vi "VI-Create XControl Dialog.vi"() -> ()   [LabVIEW 2015]
panel:
  out "exit":bool
  in  "XControl":cluster{"Folder":path, "Name":string}={"Folder"=path "D:/Experiment VIs", "Name"="New XControl"}
  in  "Create XControl":bool
  # "XControl"
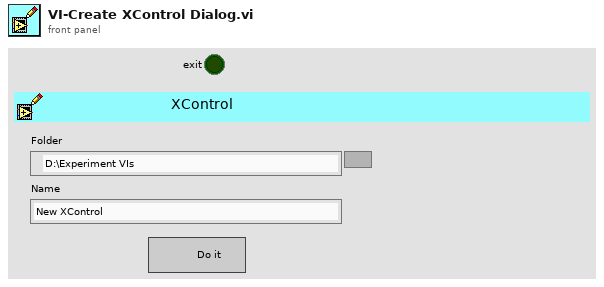
[diagram p1: front panel]
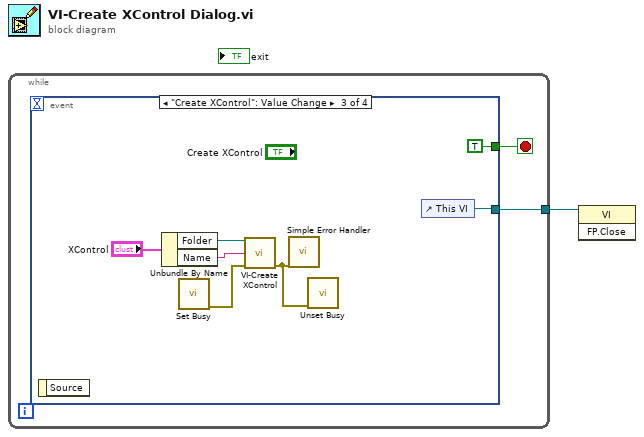
[diagram p0: block diagram]
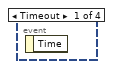
[diagram p2: hidden frame]
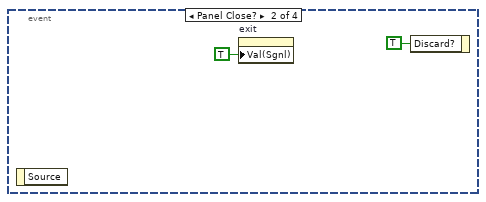
[diagram p3: hidden frame]
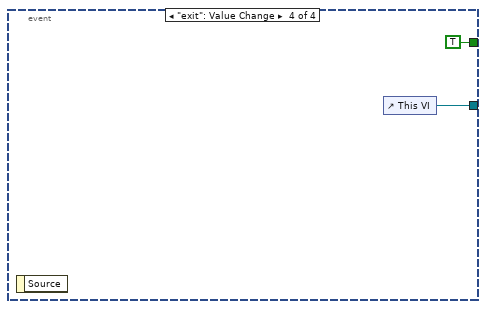
[diagram p4: hidden frame]
diagram:
  n1 = while {
    tunnel: [w3] -> w1
    stop <- w2 stop-if-true
    n2 = event shown="[2] \"Create XControl\": Value Change" {
      selector: _ -> [_ _ _ _]
      dyn-events: _ -> [_ _ _ _]
      timeout: _ -> [_ _ _ _]
      tunnel: [_ _ w8 w14] -> w3
      tunnel: [_ _ TRUE TRUE] -> w2
      event Timeout {
        n3 = event-data() -> ()  [unwired: 1 in, 1 out]
      }
      event Panel Close? {
        n4 = event-data() -> ()  [unwired: 1 in, 1 out]
        n5 = property on="exit" class="Bool (strict)"("Val(Sgnl)"=TRUE ("Value (Signaling)")) -> ()  [unwired: 2 in, 2 out]
        n6 = event-data("Discard?"=TRUE) -> ()  [unwired: 1 in, 1 out]
      }
      event "Create XControl": Value Change {
        n7 = event-data() -> ()  [unwired: 1 in, 1 out]
        n8 = Unbundle By Name("XControl") -> ("Folder"=w11:path, "Name"=w10:string)
        n9 = call <vilib>:"Set Busy.vi"() -> ("error out"=w7:errorcluster)  [unwired: 10 in, 1 out]
        n10 = call "VI-Create XControl.vi"("Folder"=w11, "Name"=w10, "error in (no error)"=w7) -> ("error out"=w6:errorcluster)  [unwired: 12 in]
        n11 = call <vilib>:"Simple Error Handler.vi"("error in (no error)"=w6) -> ()  [unwired: 4 in, 5 out]
        n12 = call <vilib>:"Unset Busy.vi"("error in (no error)"=w6) -> ()  [unwired: 10 in, 1 out]
        n13 = control-ref of="This VI"() -> (w8:refnum<vi>)
      }
      event "exit": Value Change {
        n14 = event-data() -> ()  [unwired: 1 in, 1 out]
        n15 = control-ref of="This VI"() -> (w14:refnum<vi>)
      }
    }
  }
  n16 = invoke class="VI" method="FP.Close"(reference=w1) -> ()  [unwired: 2 in, 3 out]
